vi "Step 6 - Postprocessing (Notch).vi"() -> ()   [LabVIEW 2023]
doc: "Demonstrates how to use the DFD FXP Postprocessing VI to convert the filtered signal from a fixed-point integer representation to readable engineering unit values."
uses:
  <vilib>/addons/Digital Filter Design/Design.llb/DFD IIR Notch Peak Design by Q.vi
  <vilib>/addons/Digital Filter Design/FXPModel.llb/DFD FXP Quantize Coef (Easy).vi
  <vilib>/addons/Digital Filter Design/Process.llb/DFD Filtering (PtByPt).vi
  <vilib>/Utility/VariantDataType/GetNumericFxpInfo.vi
  <vilib>/addons/Digital Filter Design/FXPSim.llb/dfd_Check Input FXP Settings.vi
  <vilib>/addons/Digital Filter Design/FXPSim.llb/dfd_Check SRate Simulation Integer Input.vi
  <vilib>/addons/Digital Filter Design/FXPSim.llb/dfd_FXP Simu.vi
  <vilib>/addons/Digital Filter Design/FXPSim.llb/DFD FXP Postprocessing (I32, 1Ch).vi
  <vilib>/addons/Digital Filter Design/_Objects.llb/DFD Quantization Sources.ctl
  <vilib>/addons/Digital Filter Design/_Objects.llb/DFD FXP Statistics Data.ctl
  <vilib>/addons/Digital Filter Design/FXPSim.llb/SimXnode/DFD FXP Simulation.xnode
  <vilib>/addons/Digital Filter Design/_Objects.llb/DFD Filter Obj.ctl
  <vilib>/addons/Digital Filter Design/_Objects.llb/DFD Filter Coef.ctl
  <vilib>/addons/Digital Filter Design/_Objects.llb/DFD Filter Structure Type Selector.ctl
  <vilib>/addons/Digital Filter Design/_Objects.llb/dfd_Internal Quantization Settings.ctl
  <vilib>/addons/Digital Filter Design/_Objects.llb/dfd_Internal Quantization Srcs.ctl
  <vilib>/addons/Digital Filter Design/_Objects.llb/DFD Coef Norm Type.ctl
  <vilib>/ptbypt/NI_PtbyPt.lvlib
  <vilib>/addons/Digital Filter Design/NI_DigFilterLicensed.lvlib
  <vilib>/addons/Digital Filter Design/NI_DigFilter_FXP.lvlib
  <vilib>/Utility/VariantDataType/VariantType.lvlib
panel:
  in  "stop":bool
  out "Signals":cluster{"sine wave":dbl, "signal out":dbl, dbl}(graph)
  in  "Test Frequency":dbl=60.0
  # "Select Help>>Show Context Help and move the cursor over the VI icon for more information."
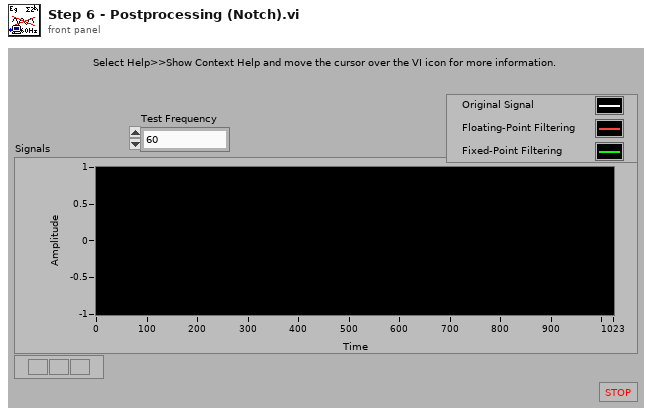
[diagram p1: front panel]
types:
  T1 = typedef "NI_DigFilterLicensed.lvlib/DFD Filter Obj.ctl" = cluster{"mSRate_Fs":dbl, "mSRate_Version":string, "mSRate_Comments":string, "mSRate_OrgCoef":T2, "mSRate_CurCoef":T2, "mSRate_Quantized?":bool, "mSRate_QCoef":T2, "mSRate_QSettings":T4[], "mSRate_Order":i32, "mSRate_Scaling":cluster{"mSRate_ScaleByPowerOf2?":bool, "mSRate_ScaleType":T6}}
  T2 = typedef "NI_DigFilterLicensed.lvlib/DFD Filter Coef.ctl" = cluster{"type":T3, "gain":dbl, "coef a (k)":dbl[], "coef b (v)":dbl[]}
  T3 = typedef "NI_DigFilterLicensed.lvlib/DFD Filter Structure Type Selector.ctl" = enum16{"Undefined", "FIR Direct Form", "FIR Direct Form Transposed", "FIR Symmetric", "FIR Antisymmetric", "IIR Direct Form I", "IIR Direct Form I Transposed", "IIR Direct Form II", "IIR Direct Form II Transposed", "IIR Cascaded Second Order Sections Form I", "IIR Cascaded Second Order Sections Form I Transposed", "IIR Cascaded Second Order Sections Form II", "IIR Cascaded Second Order Sections Form II Transposed", "Lattice Allpass (basic sections)", "Lattice Allpass (one multiplier sections)", "Lattice Allpass (normalized sections)", "Lattice AR (basic sections)", "Lattice AR (one multiplier sections)", "Lattice AR (normalized sections)", "Lattice MA (minimum phase)", "Lattice MA (maximum phase)", "Lattice ARMA (basic sections)", "Lattice ARMA (one multiplier sections)", "Lattice ARMA (normalized sections)"}
  T4 = typedef "NI_DigFilterLicensed.lvlib/dfd_Internal Quantization Settings.ctl" = cluster{"source":T5, "wl":i16, "iwl":i16, "overflow mode":enum16{"Saturation", "Wrap"}, "rounding mode":enum16{"Nearest", "Truncation"}, "signed?":bool}
  T5 = typedef "NI_DigFilterLicensed.lvlib/dfd_Internal Quantization Srcs.ctl" = u16
  T6 = typedef "NI_DigFilterLicensed.lvlib/DFD Coef Norm Type.ctl" = enum16{"No Norm", "Time Domain 1-Norm", "Time Domain 2-Norm", "Time Domain Inf-Norm"}
  T7 = cluster{"sine wave":dbl, "signal out":dbl, "Numeric":dbl}
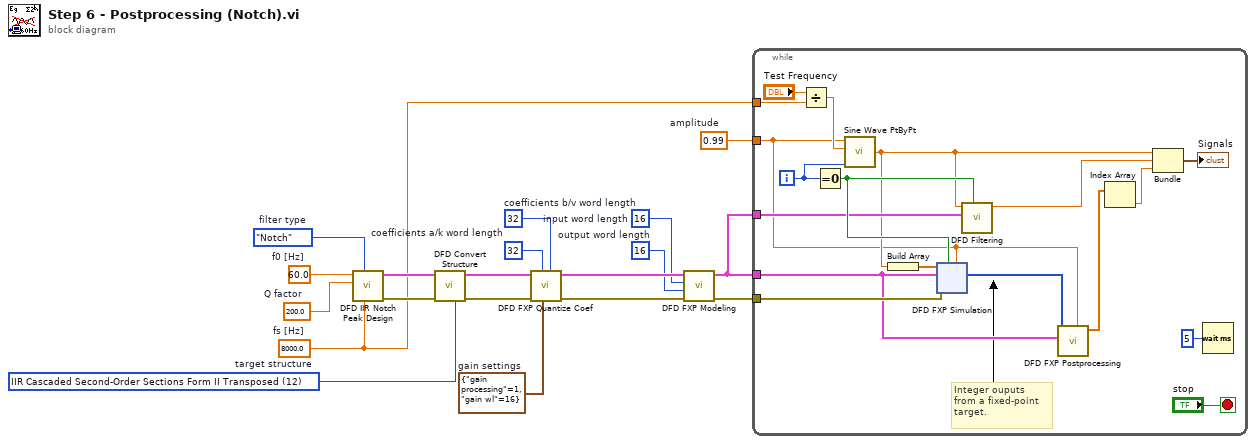
[diagram p0: block diagram]
diagram:
  w1 = i16 32  # coefficients b/v word length
  w2 = i16 32  # coefficients a/k word length
  w3 = i16 16  # output word length
  w4 = i16 16  # input word length
  w14 = u16 12 items=["FIR Direct Form"=1, "FIR Direct Form Transposed"=2, "FIR Symmetric"=3, "FIR Antisymmetric"=4, "IIR Direct Form I"=5, "IIR Direct Form I Transposed"=6, "IIR Direct Form II"=7, "IIR Direct Form II Transposed"=8, "IIR Cascaded Second-Order Sections Form I"=9, "IIR Cascaded Second-Order Sections Form I Transposed"=10, "IIR Cascaded Second-Order Sections Form II"=11, "IIR Cascaded Second-Order Sections Form II Transposed"=12, "Lattice Allpass (basic sections)"=13, "Lattice Allpass (one multiplier sections)"=14, "Lattice Allpass (normalized sections)"=15, "Lattice AR (basic sections)"=16, "Lattice AR (one multiplier sections)"=17, "Lattice AR (normalized sections)"=18, "Lattice MA (minimum phase)"=19, "Lattice MA (maximum phase)"=20, "Lattice ARMA (basic sections)"=21, "Lattice ARMA (one multiplier sections)"=22, "Lattice ARMA (normalized sections)"=23]  # target structure
  w9 = cluster{"gain processing":u16, "gain wl":i16} {"gain processing"=1, "gain wl"=16}  # gain settings
  w13 = 8000.0  # fs [Hz]
  w6 = 200.0  # Q factor
  w17 = 60.0  # f0 [Hz]
  w18 = enum16{"Notch", "Peak"}."Notch"  # filter type
  w19 = 0.99  # amplitude
  n1 = call-poly <vilib>:"DFD IIR Notch Peak Design.vi"("fs [Hz]"=w13, "filter type"=w18, "Q factor"=w6, "f0 [Hz]"=w17) -> ("error out"=w15:errorcluster, "filter out"=w16:T1)  [unwired: 1 in, 5 out]
  n2 = call <vilib>:"DFD Convert Structure.vi"("error in (no error)"=w15, "target structure"=w14, "filter in"=w16) -> ("error out"=w7:errorcluster, "filter out"=w8:T1)  [unwired: 7 out]
  n3 = call-poly <vilib>:"DFD FXP Quantize Coef.vi"("coefficients b/v word length"=w1, "gain settings"=w9, "coefficients a/k word length"=w2, "error in (no error)"=w7, "filter in"=w8) -> ("error out"=w11:errorcluster, "filter out"=w12:T1)  [unwired: 5 out]
  n4 = call <vilib>:"DFD FXP Modeling.vi"("error in (no error)"=w11, "output word length"=w3, "input word length"=w4, "filter in"=w12) -> ("error out"=w10:errorcluster, "filter out"=w5:T1)  [unwired: 3 in, 3 out]
  n5 = while {
    tunnel: w19 -> [w20]
    tunnel: w5 -> [w22]
    tunnel: w5 -> [w30]
    tunnel: w13 -> [w26]
    tunnel: w10 -> [w24]
    i -> [w34]
    stop <- "stop" stop-if-true
    # "Integer ouputs\nfrom a fixed-point\ntarget."
    n6 = Divide(x="Test Frequency", y=w26) -> (x/y=w27:dbl)
    n7 = Equal To 0?(x=w34) -> (x = 0?=w31:bool)
    n8 = call <vilib>:"Sine Wave PtByPt.vi"("time"=w34, "frequency"=w27, "amplitude"=w20) -> ("sine wave"=w28:dbl)  [unwired: 1 in]
    n9 = Build Array(w28) -> (w37:dbl[])
    n10 = xnode "DFD FXP Simulation"("input range"=w20, "init? (T)"=w31, "error in (no error)"=w24, "filter in"=w22, "signal in"=w37) -> ("integer signal out"=w23:i32[])  [unwired: 4 out]
    n11 = call-poly <vilib>:"DFD Filtering.vi"("init? (F)"=w31, "filter"=w30, "signal in"=w28) -> ("signal out"=w29:dbl)  [unwired: 1 in, 7 out]
    n12 = call-poly <vilib>:"DFD FXP Postprocessing.vi"("input range"=w20, "filter"=w22, "signal in"=w23) -> ("signal out"=w21:dbl[])  [unwired: 1 in, 7 out]
    n13 = Index Array(array=w21) -> (element=w36:dbl)  [unwired: 1 in]
    n14 = Bundle("sine wave"=w28, "signal out"=w29, "Numeric"=w36) -> (→"Signals":T7)  [unwired: 1 out]
    n15 = Wait (ms)(milliseconds to wait=u32 5) -> ()  [unwired: 1 out]
  }
